vi "IPS120_GoToField_SubVI.vi"(8 "error in (no error)":errorcluster, 11 "Mercury Targets":T1) -> (0 "error out":errorcluster)   [LabVIEW 2016, in "IPS-120.lvlib" / "IPS-120-API.lvlib"]
doc: "USE AT YOUR OWN RISK!\nThis subVI is meant to be called as a subVI of \"Mercury_GoToField.vi\", which will take care of the persistent switch for you"
uses:
  IPS-120-API.lvlib
panel:
  # "USE AT YOUR OWN RISK!\nThis subVI is meant to be called as a subVI of \"Mercury_GoToField.vi\", which will take care of the persistent switch for you"
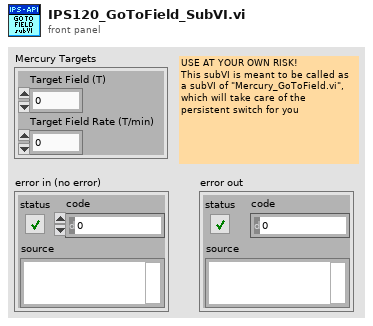
[diagram p1: front panel]
types:
  T1 = cluster{"Target Field (T)":dbl, "Target Field Rate (T/min)":dbl}
  T2 = enum16{"At Rest", "Sweeping", "Sweep Limiting", "Sweeping & Sweep Limiting"}
  T3 = typedef "IPS-120.lvlib/Read Mode 2 - Enum.ctl" = enum16{"At Rest", "Sweeping", "Sweep Limiting", "Sweeping & Sweep Limiting"}
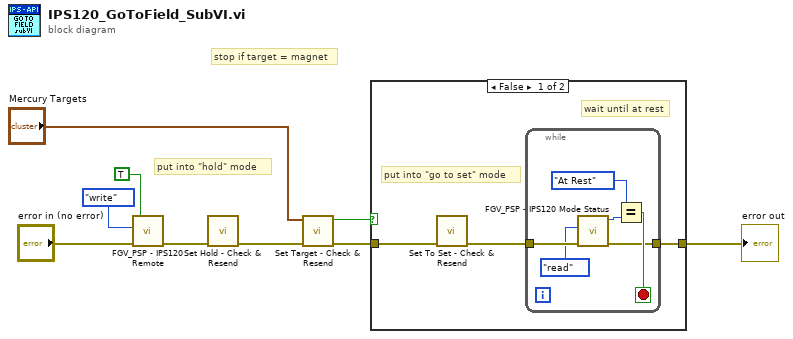
[diagram p0: block diagram]
diagram:
  # "put into \"hold\" mode"
  # "stop if target = magnet"
  n1 = call "FGV_PSP - IPS120 Remote.vi"("error in"="error in (no error)", "Function"=enum16{"write", "read"}."write", "Remote"=TRUE ("Mercury Remote")) -> ("error out"=w3:errorcluster)  [unwired: 3 in, 1 out]
  n2 = call "Set Hold - Check & Resend.vi"("error in (no error)"=w3) -> ("error out"=w2:errorcluster)  [unwired: 10 in]
  n3 = call "Set Target - Check & Resend.vi"("error in (no error)"=w2, "Mercury Targets"="Mercury Targets") -> ("error out"=w5:errorcluster, "Magnet = Target"=w4:bool)  [unwired: 8 in]
  n4 = case shown="False" w4 {
    tunnel: [w11 w19] -> w9
    tunnel: w5 -> [w10 w19]
    frame False {
      # "wait until at rest"
      # "put into \"go to set\" mode"
      n5 = call "Set To Set - Check & Resend.vi"("error in (no error)"=w10) -> ("error out"=w12:errorcluster)  [unwired: 10 in]
      n6 = while {
        tunnel: w12 -> [w17]
        tunnel: [w16] -> w11
        stop <- w18 stop-if-true
        n7 = call "FGV_PSP - IPS120 Mode Status.vi"("error in"=w17, "Function"=enum16{"write", "read"}."read") -> ("error out"=w16:errorcluster, "Mode"=w15:T3)  [unwired: 4 in]
        n8 = Equal?(x=T2."At Rest", y=w15) -> (x = y?=w18:bool)
      }
    }
    frame True {
    }
  }
  "error out" <- w9
